vi "PBI_MFA_Interface_PWM_Signals1.vi"(8 "newValue0":bool, 9 "newValue3":bool, 10 "newValue2":bool, 11 "newValue 1":bool) -> (0 "MotTstMd0":bool, 1 "MotTstMd3":bool, 2 "MotTstMd2":bool, 3 "MotTstMd1":bool)   [LabVIEW 2011]
panel:
  out "error MotorTestMode0":errorcluster
  out "error MotorTestMode 3":errorcluster
  out "error MotorTestMode2":errorcluster
  out "error MotorTestMode1":errorcluster
  out "AAABuild":i32
  in  "MintController":refnum<k7>(container)
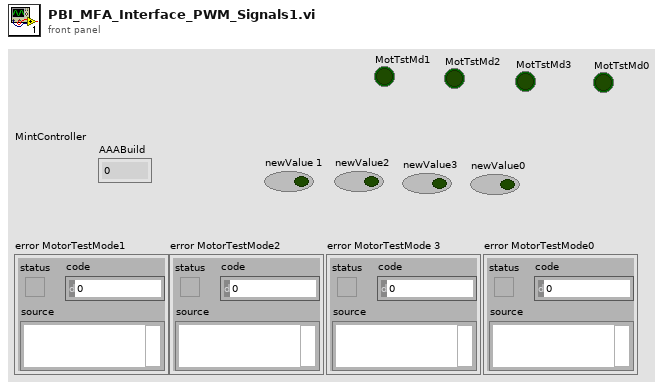
[diagram p1: front panel]
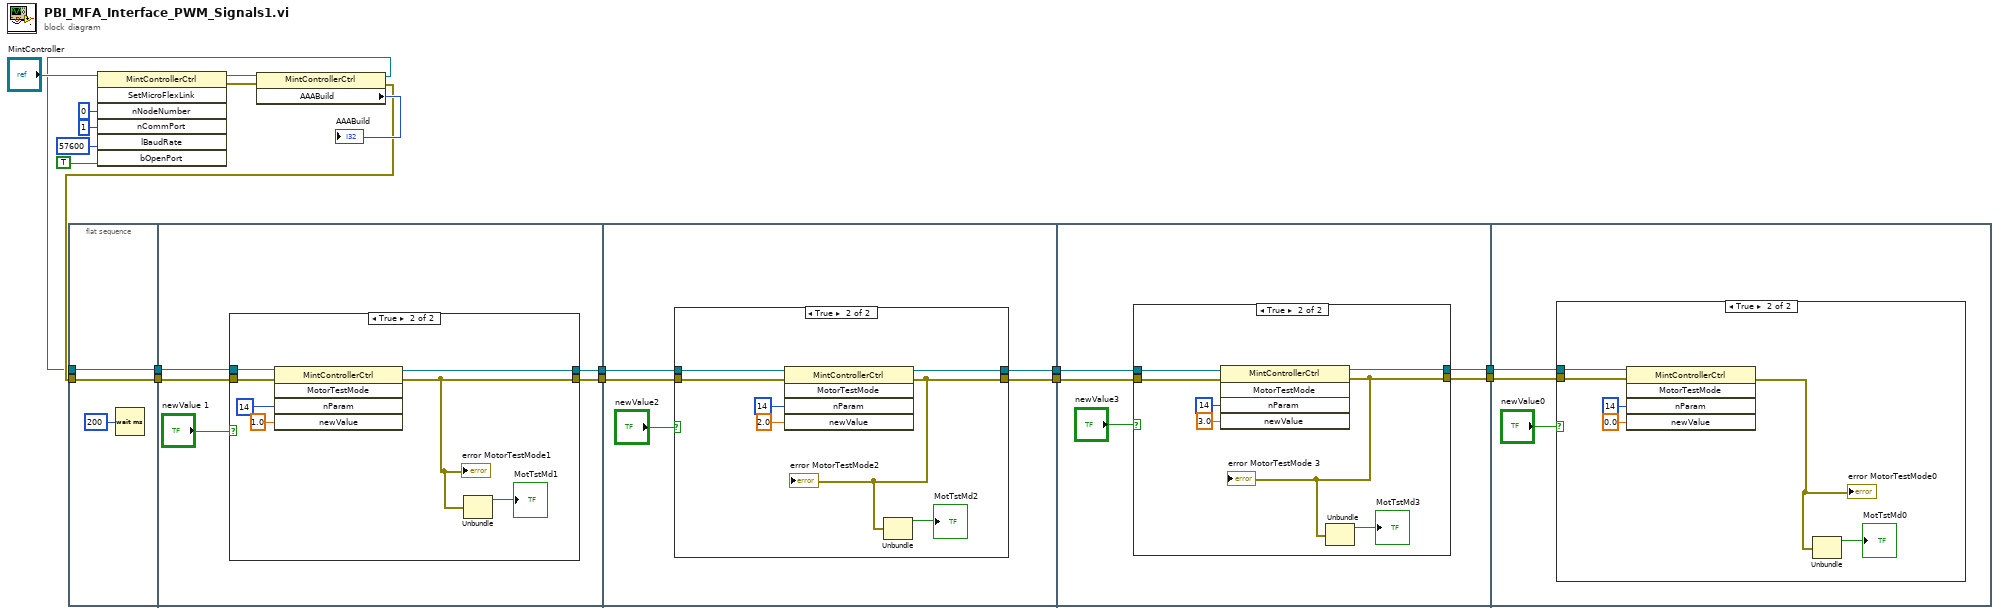
[diagram p0: block diagram]
diagram:
  n1 = flat-sequence {
    tunnel: w9 -> [w20]
    tunnel: w10 -> [w21]
    tunnel: [w21] -> w8
    tunnel: [w20] -> w7
    tunnel: w8 -> [w26]
    tunnel: w7 -> [w25]
    tunnel: [w24] -> w6
    tunnel: [w23] -> w5
    tunnel: w6 -> [w39]
    tunnel: w5 -> [w40]
    tunnel: [w38] -> w4
    tunnel: [w37] -> w3
    tunnel: w4 -> [w53]
    tunnel: w3 -> [w54]
    tunnel: [w52] -> w2
    tunnel: [w51] -> w1
    tunnel: w2 -> [w65]
    tunnel: w1 -> [w66]
    frame #0 {
      n2 = Wait (ms)(milliseconds to wait=u32 200) -> ()  [unwired: 1 out]
    }
    frame #1 {
      n3 = case shown="True" "newValue 1" {
        tunnel: w26 -> [w27 w34]
        tunnel: w25 -> [w28 w33]
        tunnel: [w27 w30] -> w24
        tunnel: [w28 w32] -> w23
        frame False {
        }
        frame True {
          n4 = invoke class="MintControllerCtrl" method="MotorTestMode"(reference=w33, error in=w34, "nParam"=i16 14 ("nAxis"), "newValue"=sgl 1.0) -> (reference out=w32:refnum<k7>, error out=w30:errorcluster)  [unwired: 1 in, 3 out]
          "error MotorTestMode1" <- w30
          n5 = Unbundle(w30) -> ("status"=→"MotTstMd1":bool)  [unwired: 2 out]
        }
      }
    }
    frame #2 {
      n6 = case shown="True" "newValue2" {
        tunnel: w40 -> [w42 w49]
        tunnel: w39 -> [w41 w48]
        tunnel: [w41 w43] -> w38
        tunnel: [w42 w45] -> w37
        frame False {
        }
        frame True {
          n7 = invoke class="MintControllerCtrl" method="MotorTestMode"(reference=w49, error in=w48, "nParam"=i16 14, "newValue"=sgl 2.0) -> (reference out=w45:refnum<k7>, error out=w43:errorcluster)  [unwired: 1 in, 3 out]
          "error MotorTestMode2" <- w43
          n8 = Unbundle(w43) -> ("status"=→"MotTstMd2":bool)  [unwired: 2 out]
        }
      }
    }
    frame #3 {
      n9 = case shown="True" "newValue3" {
        tunnel: w54 -> [w56 w63]
        tunnel: w53 -> [w55 w62]
        tunnel: [w55 w57] -> w52
        tunnel: [w56 w60] -> w51
        frame False {
        }
        frame True {
          n10 = invoke class="MintControllerCtrl" method="MotorTestMode"(reference=w63, error in=w62, "nParam"=i16 14 ("nAxis"), "newValue"=sgl 3.0) -> (reference out=w60:refnum<k7>, error out=w57:errorcluster)  [unwired: 1 in, 3 out]
          "error MotorTestMode 3" <- w57
          n11 = Unbundle(w57) -> ("status"=→"MotTstMd3":bool)  [unwired: 2 out]
        }
      }
    }
    frame #4 {
      n12 = case shown="True" "newValue0" {
        tunnel: w66 -> [_ w72]
        tunnel: w65 -> [_ w71]
        frame False {
        }
        frame True {
          n13 = invoke class="MintControllerCtrl" method="MotorTestMode"(reference=w72, error in=w71, "nParam"=i16 14 ("nAxis"), "newValue"=sgl 0.0) -> (error out=w67:errorcluster)  [unwired: 1 in, 4 out]
          "error MotorTestMode0" <- w67
          n14 = Unbundle(w67) -> ("status"=→"MotTstMd0":bool)  [unwired: 2 out]
        }
      }
    }
  }
  n15 = invoke class="MintControllerCtrl" method="SetMicroFlexLink"(reference="MintController", "nNodeNumber"=i16 0, "nCommPort"=i16 1, "lBaudRate"=57600, "bOpenPort"=TRUE) -> (reference out=w18:refnum<k7>, error out=w12:errorcluster)  [unwired: 2 in, 5 out]
  n16 = property class="MintControllerCtrl"(reference=w18, error in=w12) -> (reference out=w9:refnum<k7>, error out=w10:errorcluster, "AAABuild"=→"AAABuild":i32)
